vi "TruncatetoMapEdge.vi"(8 "dx":dbl, 11 "dy":dbl) -> (0 "Target X":dbl, 3 "Target Y":dbl)   [LabVIEW 2011]
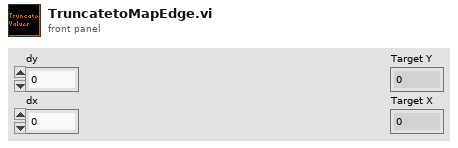
[diagram p1: front panel]
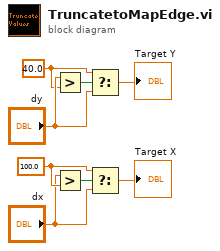
[diagram p0: block diagram]
diagram:
  w4 = 100.0 ("t")
  w6 = 40.0 ("t")
  n1 = Greater?(x="dy", y=w6) -> (0:w8:bool)
  n2 = Greater?(x="dx", y=w4) -> (0:w5:bool)
  n3 = Select(t=w6, s=w8, f="dy") -> (s? t:f=→"Target Y":dbl)
  n4 = Select(t=w4, s=w5, f="dx") -> (s? t:f=→"Target X":dbl)
